vi "CmdExe.Run VI with Timeout and Abort.vi"(7 "Close Ref":bool=TRUE, 8 "error in (no error)":errorcluster, 10 "Timeout ms(-1)":i32=-1, 11 "VI Refnum":refnum<vi>) -> (0 "error out":errorcluster, 2 "Timeout":bool, 3 "Abort":bool)   [LabVIEW 2018]
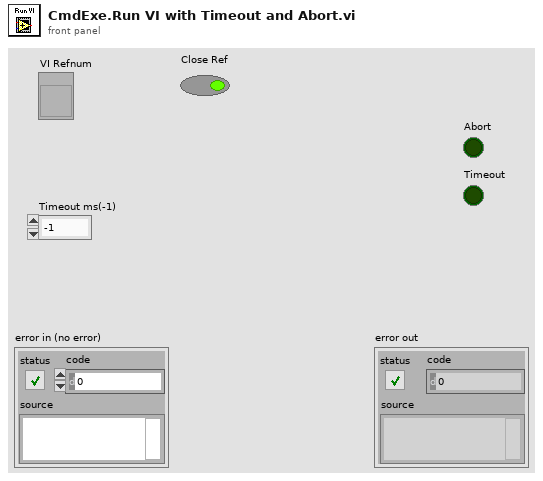
[diagram p1: front panel]
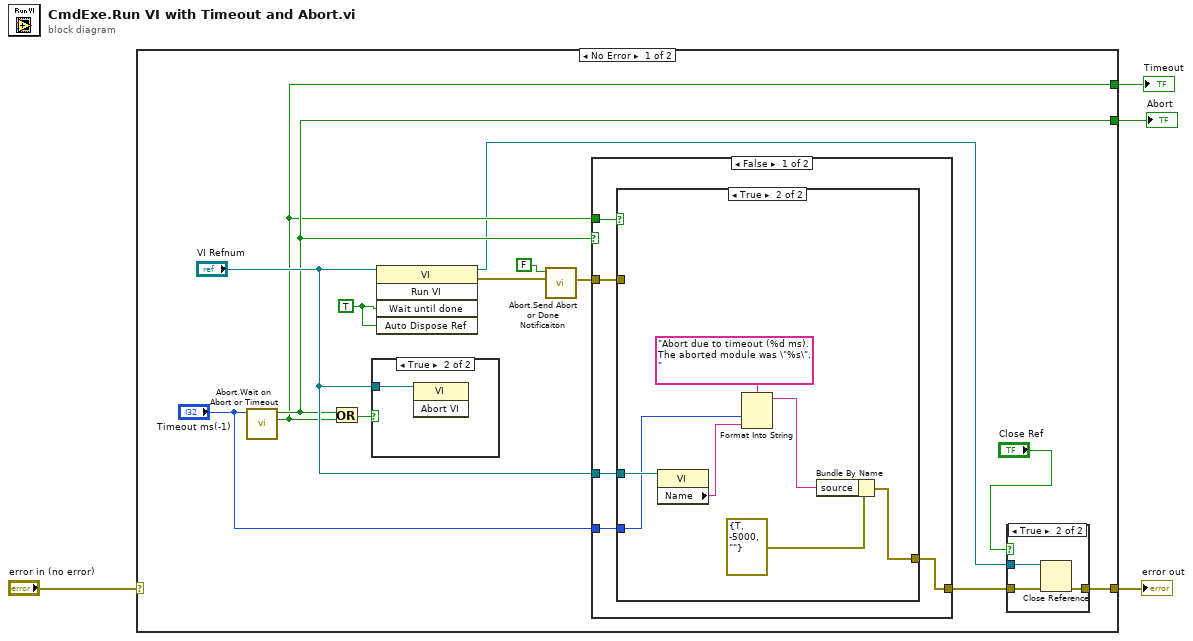
[diagram p0: block diagram]
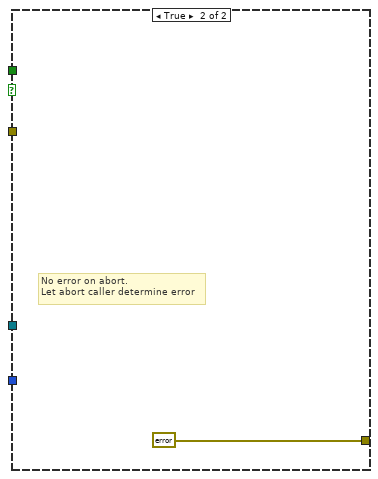
[diagram p4: hidden frame]
diagram:
  n1 = case shown="No Error" "error in (no error)" {
    selector: "error in (no error)" -> [_ w37]
    tunnel: [w7 w37] -> w3
    tunnel: [w11 _] -> w2
    tunnel: [w10 _] -> w1
    frame No Error {
      w17 = TRUE ("Wait Until Done")
      n2 = call "Abort.Wait on Abort or Timeout.vi"("Timeout ms (-1)"="Timeout ms(-1)") -> ("Timeout"=w10:bool, "Abort"=w11:bool)  [unwired: 9 in]
      n3 = Or(x=w11, y=w10) -> (x .or. y?=w14:bool)
      n4 = case shown="True" w14 {
        tunnel: "VI Refnum" -> [_ w36]
        frame False {
        }
        frame True {
          n5 = invoke class="VI" method="Abort VI"(reference=w36) -> ()  [unwired: 2 in, 3 out]
        }
      }
      n6 = invoke class="VI" method="Run VI"(reference="VI Refnum", "Wait until done"=w17, "Auto Dispose Ref"=w17) -> (reference out=w6:refnum<vi>, error out=w15:errorcluster)  [unwired: 2 in, 3 out]
      n7 = call "Abort.Send Abort or Done Notificaiton.vi"("Error"=w15, "Abort(T)/Done(F)"=FALSE) -> ("error out"=w13:errorcluster)  [unwired: 9 in]
      n8 = case shown="False" w11 {
        tunnel: w10 -> [w26 _]
        tunnel: [w24 errorcluster {"status"=FALSE, "code"=0, "source"=""} ("error constant")] -> w8
        tunnel: w13 -> [w23 _]
        tunnel: "VI Refnum" -> [w25 _]
        tunnel: "Timeout ms(-1)" -> [w22 _]
        frame False {
          n9 = case shown="True" w26 {
            tunnel: w25 -> [_ w34]
            tunnel: [w27 w28] -> w24
            tunnel: w23 -> [w27 _]
            tunnel: w22 -> [_ w31]
            frame False {
              # "No abort or timeout"
            }
            frame True {
              n10 = property class="VI"(reference=w34) -> ("Name"=w32:string)  [unwired: 1 in, 2 out]
              n11 = Format Into String(format string="Abort due to timeout (%d ms).  The aborted module was \"%s\".", w31, w32) -> (resulting string=w29:string)  [unwired: 2 in, 1 out]
              n12 = Bundle By Name(cluster=errorcluster {"status"=TRUE, "code"=-5000, "source"=""} ("error constant"), "source"=w29) -> (w28:errorcluster)
            }
          }
        }
        frame True {
          # "No error on abort.\nLet abort caller determine error"
        }
      }
      n13 = case shown="True" "Close Ref" {
        tunnel: w8 -> [w18 w21]
        tunnel: [w18 w20] -> w7
        tunnel: w6 -> [_ w19]
        frame False {
        }
        frame True {
          n14 = Close Reference(reference=w19, error in (no error)=w21) -> (error out=w20:errorcluster)
        }
      }
    }
    frame Error {
    }
  }
  "error out" <- w3
  "Abort" <- w2
  "Timeout" <- w1
